vi "write_Xy.vi"(8 "error in (no error)":errorcluster, 10 "Xy":dbl[][](array[numeric]), 11 "Lars in":refnum<class "Lars.lvclass">) -> (0 "error out":errorcluster, 3 "Lars out":refnum<class "Lars.lvclass">)   [LabVIEW 2020, in "Lars.lvclass"]
uses:
  Lars.lvclass
  Lars.lvclass/Lars.ctl
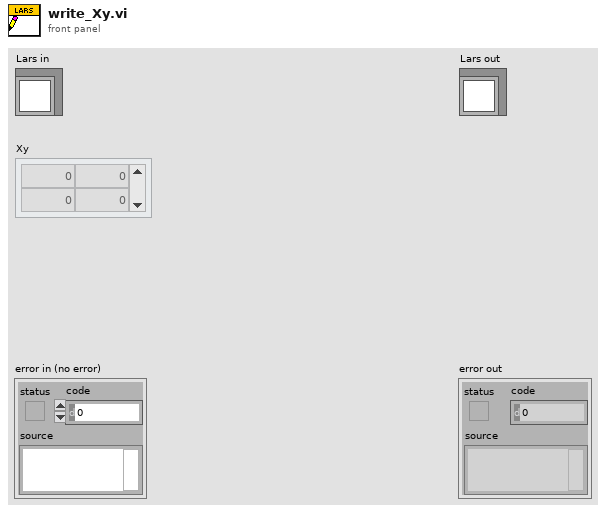
[diagram p1: front panel]
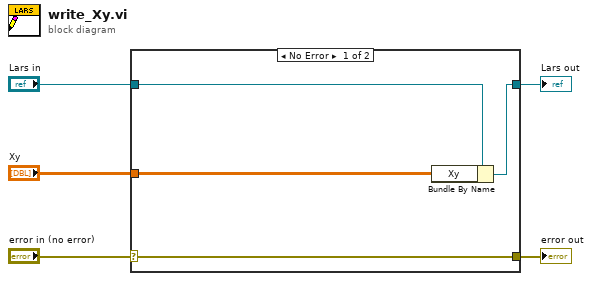
[diagram p0: block diagram]
diagram:
  n1 = case shown="No Error" "error in (no error)" {
    selector: "error in (no error)" -> [w9 w10]
    tunnel: [w9 w10] -> w4
    tunnel: [w7 w11] -> w2
    tunnel: "Lars in" -> [w8 w11]
    tunnel: "Xy" -> [w6 _]
    frame No Error {
      n2 = Bundle By Name(cluster=w8, "Xy"=w6) -> (w7:refnum<class "Lars.lvclass">)
    }
    frame Error {
    }
  }
  "error out" <- w4
  "Lars out" <- w2
